vi "control_instruments.vi"(2 "error in (no error)":errorcluster, 3 "Data in":string[](array[string])) -> (0 "error out (no error)":errorcluster, 1 "Measurement Data":string[](array[string]))   [LabVIEW 2011]
doc: "Control_instruments\n\nThis Vi will let those instruments that are in need of update be updated. Some instruments will always require an update even if the current settings are the same as the new settings, this is called Forced Update, and can be set up in the front panel."
panel:
  out "x-y":u32
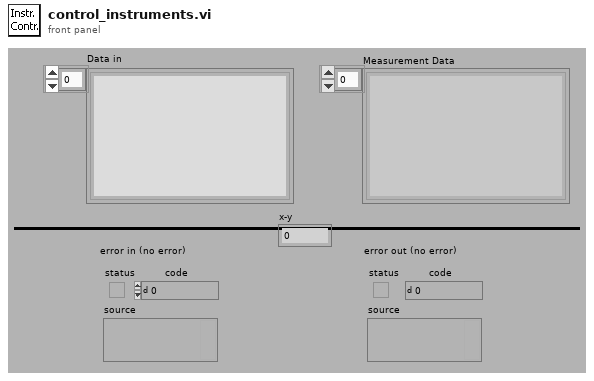
[diagram p1: front panel]
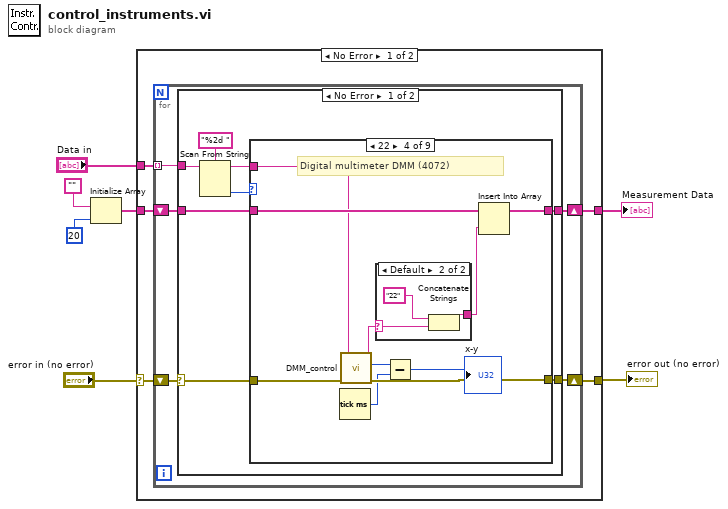
[diagram p0: block diagram]
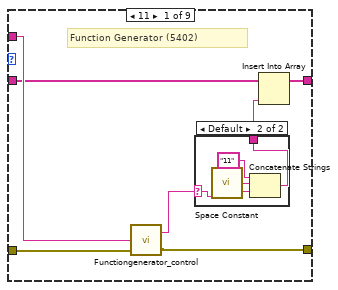
[diagram p2: hidden frame]
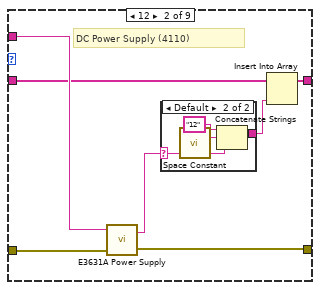
[diagram p4: hidden frame]
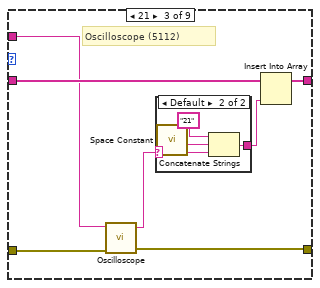
[diagram p6: hidden frame]
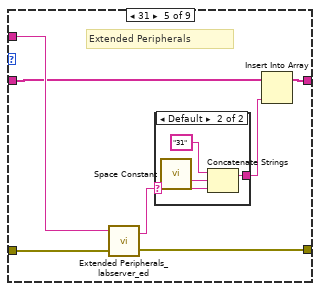
[diagram p9: hidden frame]
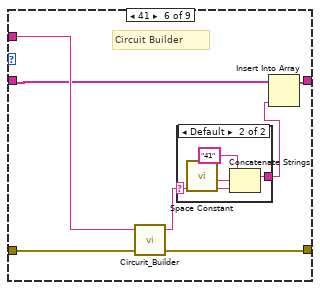
[diagram p11: hidden frame]
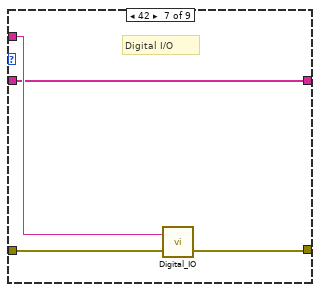
[diagram p13: hidden frame]
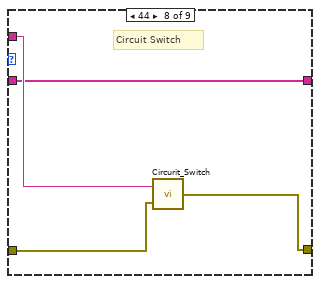
[diagram p14: hidden frame]
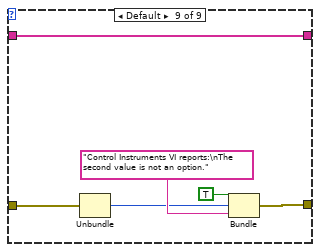
[diagram p15: hidden frame]
diagram:
  n1 = Initialize Array("", 20) -> (w5:string[])
  n2 = case shown="No Error" "error in (no error)" {
    selector: "error in (no error)" -> [w9 w116]
    tunnel: w5 -> [w12 w117]
    tunnel: [w10 w116] -> w3
    tunnel: [w11 w117] -> w4
    tunnel: "Data in" -> [w8 _]
    frame No Error {
      n3 = for {
        shift-right: [w17] -> w11
        shift-left: w12 -> [w15]
        shift-right: [w16] -> w10
        shift-left: w9 -> [w13]
        tunnel: w8 -> [w14] mode=indexing
        n4 = case shown="No Error" w13 {
          selector: w13 -> [w18 w114]
          tunnel: [w25 w115] -> w17
          tunnel: [w24 w114] -> w16
          tunnel: w15 -> [w23 w115]
          tunnel: w14 -> [w21 _]
          frame No Error {
            n5 = Scan From String(format string="%2d ", input string=w21) -> (remaining string=w20:string, output 1=w19:i32)  [unwired: 3 in, 2 out]
            n6 = case shown="22" w19 {
              tunnel: w20 -> [w31 w43 w50 w68 w82 w94 w103 w105 _]
              tunnel: w23 -> [w27 w40 w53 w71 w78 w90 w101 w104 w108]
              tunnel: [w28 w39 w54 w70 w77 w89 w101 w104 w108] -> w25
              tunnel: w18 -> [w32 w44 w56 w66 w81 w93 w100 w107 w110]
              tunnel: [w30 w42 w55 w65 w80 w92 w102 w106 w109] -> w24
              frame 11 {
                # "Function Generator (5402)"
                n7 = call "Functiongenerator_control.vi"("error in (no error)"=w32, "Data in"=w31) -> ("error out (no error)"=w30:errorcluster, "Data Out"=w26:string)  [unwired: 1 in]
                n8 = case shown="Default" w26 {
                  selector: w26 -> [w33 w35]
                  tunnel: [w33 w36] -> w29
                  frame "" {
                  }
                  frame Default {
                    n9 = call <vilib>:"Space Constant.vi"() -> ("String"=w34:string)
                    n10 = Concatenate Strings("11", w34, w35) -> (w36:string)
                  }
                }
                n11 = Insert Into Array(array=w27, new element=w29) -> (w28:string[])  [unwired: 1 in]
              }
              frame 12 {
                # "DC Power Supply (4110)"
                n12 = call "E3631A Power Supply.vi"("error in (no error)"=w44, "Data input"=w43) -> ("error out (no error)"=w42:errorcluster, "Data output"=w38:string)  [unwired: 1 in]
                n13 = case shown="Default" w38 {
                  selector: w38 -> [w45 w47]
                  tunnel: [w45 w48] -> w41
                  frame "" {
                  }
                  frame Default {
                    n14 = call <vilib>:"Space Constant.vi"() -> ("String"=w46:string)
                    n15 = Concatenate Strings("12", w46, w47) -> (w48:string)
                  }
                }
                n16 = Insert Into Array(array=w40, new element=w41) -> (w39:string[])  [unwired: 1 in]
              }
              frame 21 {
                # "Oscilloscope (5112)"
                n17 = call "Oscilloscope.vi"("error in (no error)"=w56, "Data In"=w50) -> ("error out (no error)"=w55:errorcluster, "Data out"=w51:string)  [unwired: 3 in]
                n18 = case shown="Default" w51 {
                  selector: w51 -> [w57 w59]
                  tunnel: [w57 w60] -> w52
                  frame "" {
                  }
                  frame Default {
                    n19 = call <vilib>:"Space Constant.vi"() -> ("String"=w58:string)
                    n20 = Concatenate Strings("21", w58, w59) -> (w60:string)
                  }
                }
                n21 = Insert Into Array(array=w53, new element=w52) -> (w54:string[])  [unwired: 1 in]
              }
              frame 22 {
                # "Digital multimeter DMM (4072)"
                n22 = Tick Count (ms)() -> (millisecond timer value=w64:u32)
                n23 = call "DMM_control.vi"("Data in"=w68, "error in"=w66) -> ("Data out"=w67:string, "millisecond timer value"=w63:u32, "error out"=w65:errorcluster)  [unwired: 4 in]
                n24 = case shown="Default" w67 {
                  selector: w67 -> [w72 w74]
                  tunnel: [w72 w75] -> w69
                  frame "" {
                  }
                  frame Default {
                    n25 = Concatenate Strings("22", w74) -> (w75:string)
                  }
                }
                n26 = Subtract(x=w63, y=w64) -> (x-y=→"x-y":u32)
                n27 = Insert Into Array(array=w71, new element=w69) -> (w70:string[])  [unwired: 1 in]
              }
              frame 31 {
                # "Extended Peripherals"
                n28 = call "Extended Peripherals_labserver_ed.vi"("error in (no error)"=w81, "Command In"=w82) -> ("error out (no error)"=w80:errorcluster, "DataOut"=w76:string)  [unwired: 1 in]
                n29 = case shown="Default" w76 {
                  selector: w76 -> [w83 w85]
                  tunnel: [w83 w86] -> w79
                  frame "" {
                  }
                  frame Default {
                    n30 = call <vilib>:"Space Constant.vi"() -> ("String"=w84:string)
                    n31 = Concatenate Strings("31", w84, w85) -> (w86:string)
                  }
                }
                n32 = Insert Into Array(array=w78, new element=w79) -> (w77:string[])  [unwired: 1 in]
              }
              frame 41 {
                # "Circuit Builder"
                n33 = call "Circurit_Builder.vi"("error in (no error)"=w93, "Data in"=w94) -> ("error out (no error)"=w92:errorcluster, "DataOut"=w88:string)  [unwired: 2 in]
                n34 = case shown="Default" w88 {
                  selector: w88 -> [w95 w97]
                  tunnel: [w95 w98] -> w91
                  frame "" {
                  }
                  frame Default {
                    n35 = call <vilib>:"Space Constant.vi"() -> ("String"=w96:string)
                    n36 = Concatenate Strings("41", w96, w97) -> (w98:string)
                  }
                }
                n37 = Insert Into Array(array=w90, new element=w91) -> (w89:string[])  [unwired: 1 in]
              }
              frame 42 {
                # "Digital I/O"
                n38 = call "Digital_IO.vi"("error in"=w100, "Data in"=w103) -> ("error out (no error)"=w102:errorcluster)  [unwired: 1 in]
              }
              frame 44 {
                # "Circuit Switch"
                n39 = call "Circurit_Switch.vi"("error in (no error)"=w107, "Data in"=w105) -> ("error out (no error)"=w106:errorcluster)
              }
              frame Default {
                n40 = Unbundle(w110) -> ("code"=w111:i32)  [unwired: 2 out]
                n41 = Bundle("status"=TRUE, "code"=w111, "Control Instruments VI reports:\nThe second value is not an option.") -> (w109:cluster{"status":bool, "code":i32, string})  [unwired: 1 in]
              }
            }
          }
          frame Error {
            # "An error has occoured!\nHalt execution!"
          }
        }
      }
    }
    frame Error {
    }
  }
  "Measurement Data" <- w4
  "error out (no error)" <- w3
